vi "lockin_controller.vi"(10 "Numerical Argument":dbl, 11 "Command":T1(ring)=enum."Get Amplitude") -> (3 "Response":string)   [LabVIEW 2021]
panel:
  # "LOCKIN AMPLIFIER CONTROLLER"
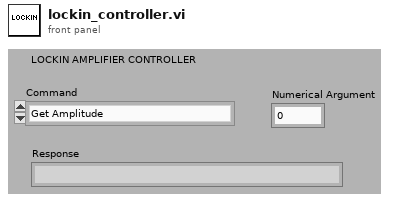
[diagram p1: front panel]
types:
  T1 = enum16{"Set Amplitude", "Get Amplitude", "Set Frequency", "Get Frequency", "Set Harmonic", "Get Harmonic", "Set Phase", "Get Phase", "Auto Phase", "Add to Phase", "Autogain", "Set Time Constant", "Get Time Constant", "Set Sensitivity", "Get Sensitivity", "Set Input A", "Set Input A-B", "Get Input Setting", "Set Offset", "Get Offset"}
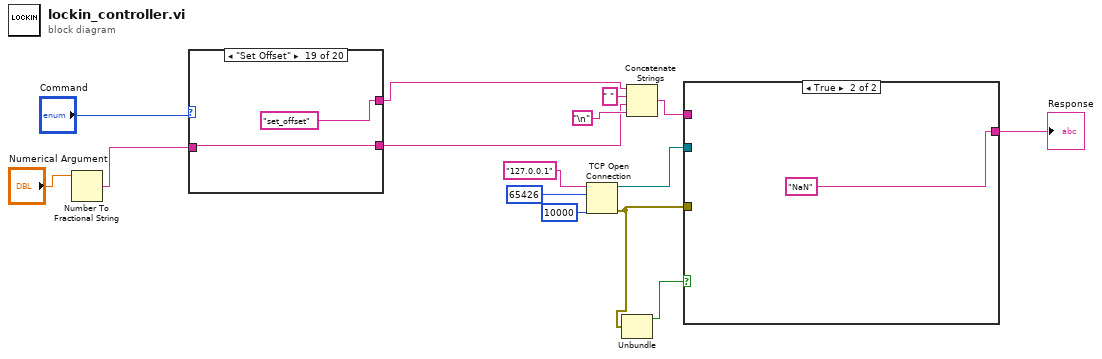
[diagram p0: block diagram]
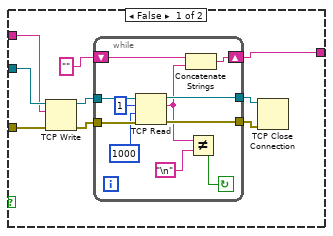
[diagram p2: hidden frame]
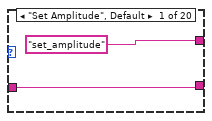
[diagram p3: hidden frame]
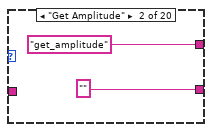
[diagram p4: hidden frame]
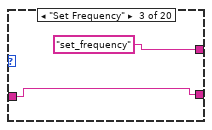
[diagram p5: hidden frame]
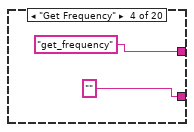
[diagram p6: hidden frame]
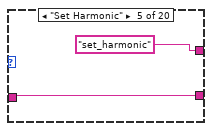
[diagram p7: hidden frame]
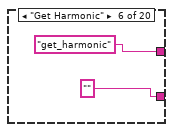
[diagram p8: hidden frame]
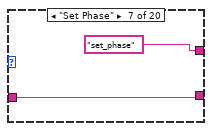
[diagram p9: hidden frame]
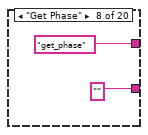
[diagram p10: hidden frame]
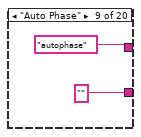
[diagram p11: hidden frame]
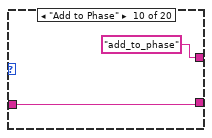
[diagram p12: hidden frame]
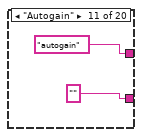
[diagram p13: hidden frame]
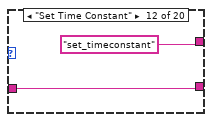
[diagram p14: hidden frame]
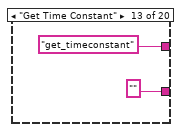
[diagram p15: hidden frame]
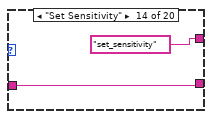
[diagram p16: hidden frame]
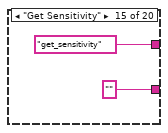
[diagram p17: hidden frame]
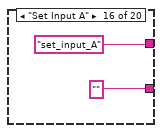
[diagram p18: hidden frame]
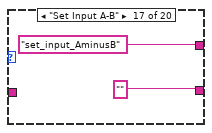
[diagram p19: hidden frame]
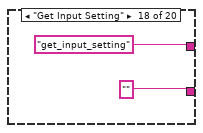
[diagram p20: hidden frame]
diagram:
  n1 = Number To Fractional String(number="Numerical Argument") -> (F-format string=w6:string)  [unwired: 3 in]
  n2 = case shown="\"Set Offset\"" "Command" {
    tunnel: ["set_amplitude" ("data in") "get_amplitude" ("data in") "set_frequency" ("data in") "get_frequency" ("data in") "set_harmonic" ("data in") "get_harmonic" ("data in") "set_phase" ("data in") "get_phase" ("data in") "autophase" ("data in") "add_to_phase" ("data in") "autogain" ("data in") "set_timeconstant" ("data in") "get_timeconstant" ("data in") "set_sensitivity" ("data in") "get_sensitivity" ("data in") "set_input_A" ("data in") "set_input_AminusB" ("data in") "get_input_setting" ("data in") "set_offset" ("data in") "get_offset" ("data in")] -> w4
    tunnel: [w16 "" ("string") w20 "" ("string") w24 "" ("string") w28 "" ("string") "" ("string") w34 "" ("string") w39 "" ("string") w42 "" ("string") "" ("string") "" ("string") "" ("string") w52 "" ("string")] -> w7
    tunnel: w6 -> [w16 _ w20 _ w24 _ w28 _ _ w34 _ w39 _ w42 _ _ _ _ w52 _]
    frame "Set Amplitude", Default {
    }
    frame "Get Amplitude" {
    }
    frame "Set Frequency" {
    }
    frame "Get Frequency" {
    }
    frame "Set Harmonic" {
    }
    frame "Get Harmonic" {
    }
    frame "Set Phase" {
    }
    frame "Get Phase" {
    }
    frame "Auto Phase" {
    }
    frame "Add to Phase" {
    }
    frame "Autogain" {
    }
    frame "Set Time Constant" {
    }
    frame "Get Time Constant" {
    }
    frame "Set Sensitivity" {
    }
    frame "Get Sensitivity" {
    }
    frame "Set Input A" {
    }
    frame "Set Input A-B" {
    }
    frame "Get Input Setting" {
    }
    frame "Set Offset" {
    }
    frame "Get Offset" {
    }
  }
  n3 = TCP Open Connection(address="127.0.0.1", remote port or service name=u16 65426, timeout ms (60000)=10000) -> (connection ID=w13:refnum<k5>, error out=w3:errorcluster)  [unwired: 2 in]
  n4 = Unbundle(w3) -> ("status"=w2:bool)  [unwired: 2 out]
  n5 = Concatenate Strings(w4, " " ("string"), w7, "\n") -> (w11:string)
  n6 = case shown="True" w2 {
    tunnel: w13 -> [w64 _]
    tunnel: [w58 "NaN"] -> w12
    tunnel: w11 -> [w57 _]
    tunnel: w3 -> [w56 _]
    frame False {
      n7 = TCP Write(connection ID=w64, data in=w57, error in (no error)=w56) -> (connection ID out=w62:refnum<k5>, error out=w63:errorcluster)  [unwired: 1 in, 1 out]
      n8 = while {
        tunnel: w63 -> [w75]
        tunnel: w62 -> [w74]
        tunnel: [w73] -> w61
        tunnel: [w72] -> w60
        shift-right: [w68] -> w58
        shift-left: "" ("string") -> [w69]
        stop <- w67 continue-if-true
        n9 = TCP Read(connection ID=w74, bytes to read=1, error in (no error)=w75, 9:1000 ("timeout ms (25000)")) -> (connection ID out=w72:refnum<k5>, data out=w66:string, error out=w73:errorcluster)  [unwired: 1 in]
        n10 = Concatenate Strings(w69, w66) -> (w68:string)
        n11 = Not Equal?(x=w66, y="\n") -> (x != y?=w67:bool)
      }
      n12 = TCP Close Connection(connection ID=w60, error in (no error)=w61) -> ()  [unwired: 1 in, 2 out]
    }
    frame True {
    }
  }
  "Response" <- w12
